vi "Connect.vi"   [LabVIEW 2020, in "ORM_API.lvlib"]
uses:
  ORM_API.lvlib
  <vilib>/Viviota/shared/ORM_DBC_Mssql.lvlibp/DBC.lvclass
  <vilib>/Viviota/shared/ORM_DBC_MySql.lvlibp/DBC.lvclass
  <vilib>/Viviota/shared/ORM_DBC_Npgsql.lvlibp/DBC.lvclass
  <vilib>/Viviota/shared/ORM_DBC_Odbc.lvlibp/DBC.lvclass
  <vilib>/Viviota/shared/ORM_DBC_Sqlite.lvlibp/DBC.lvclass
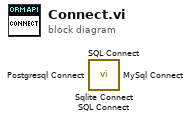
[diagram p0: block diagram]
diagram:
  n1 = call <vilib>:"Sqlite Connect.vi"() -> ()  [unwired: 10 in, 2 out]
  n2 = call <vilib>:"SQL Connect.vi"() -> ()  [unwired: 10 in, 2 out]
  n3 = call <vilib>:"Postgresql Connect.vi"() -> ()  [unwired: 10 in, 2 out]
  n4 = call <vilib>:"MySql Connect.vi"() -> ()  [unwired: 10 in, 2 out]
  n5 = call <vilib>:"SQL Connect.vi"() -> ()  [unwired: 10 in, 2 out]
